vi "Read port.vi"(8 "error in (no error)":errorcluster, 11 "ServerListener in":refnum<class "ServerListener.lvclass">) -> (0 "error out":errorcluster, 2 "port":u16=6341, 3 "ServerListener out":refnum<class "ServerListener.lvclass">)   [LabVIEW 2016, in "ServerListener.lvlib" / "ServerListener.lvclass"]
uses:
  ServerListener.lvclass
  ServerListener.lvclass/ServerListener.ctl
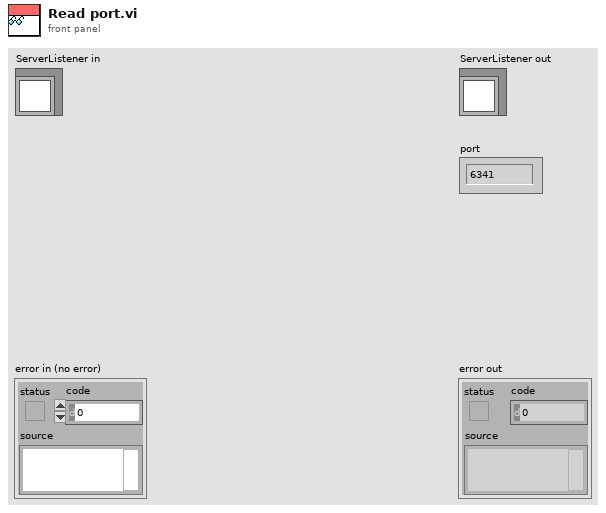
[diagram p1: front panel]
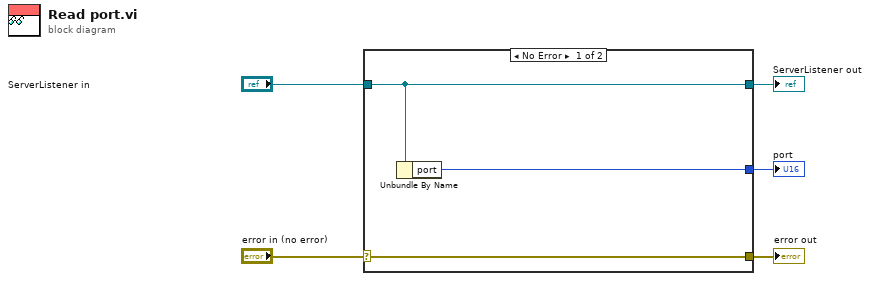
[diagram p0: block diagram]
diagram:
  n1 = case shown="No Error" "error in (no error)" {
    selector: "error in (no error)" -> [w8 w9]
    tunnel: [w8 w9] -> w4
    tunnel: [w7 w10] -> w2
    tunnel: "ServerListener in" -> [w7 w10]
    tunnel: [w6 _] -> w1
    frame No Error {
      n2 = Unbundle By Name(w7) -> ("port"=w6:u16)
    }
    frame Error {
    }
  }
  "error out" <- w4
  "ServerListener out" <- w2
  "port" <- w1
